vi "Convert-U64-to-String.vi"(8 "error in":errorcluster, 10 "Array (U64) in":u64[](array[numeric]) format="%.0x", 11 "Title":string="FIFO Dump") -> (0 "error out":errorcluster, 3 "String out":string)   [LabVIEW 2018]
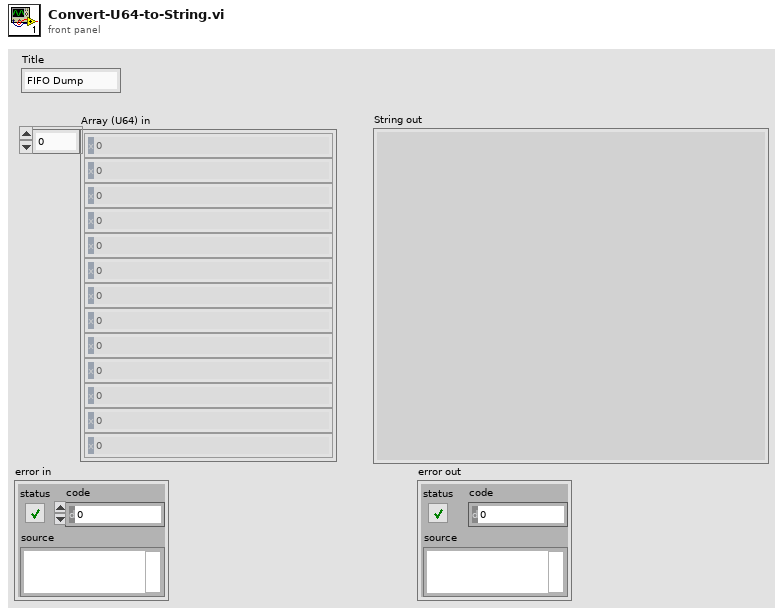
[diagram p1: front panel]
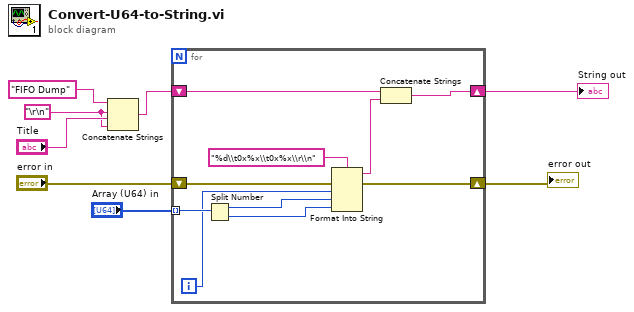
[diagram p0: block diagram]
diagram:
  w3 = "\r\n"
  n1 = Concatenate Strings("FIFO Dump", w3, "Title", w3) -> (w5:string)
  n2 = for {
    tunnel: "Array (U64) in" -> [w18] mode=indexing
    shift-right: [w14] -> w7
    shift-left: w5 -> [w16]
    shift-right: [w10] -> w2
    shift-left: "error in" -> [w9]
    i -> [w13]
    n3 = Split Number(x=w18) -> (hi(x)=w12:u32, lo(x)=w11:u32)
    n4 = Format Into String(format string="%d\\t0x%x\\t0x%x\\r\\n", error in=w9, w13, w12, w11) -> (resulting string=w15:string, error out=w10:errorcluster)  [unwired: 1 in]
    n5 = Concatenate Strings(w16, w15) -> (w14:string)
  }
  "String out" <- w7
  "error out" <- w2
